vi "checkSettled.vi"(8 "error in (no error)":errorcluster, 11 "Model in":refnum<class "Model.lvclass">) -> (0 "error out":errorcluster, 2 "settledIsTrue":bool, 3 "Model out":refnum<class "Model.lvclass">)   [LabVIEW 2015, in "Model.lvclass"]
uses:
  Model.lvclass
  Model.lvclass/Model.ctl
  ApplicationElements/SystemController/SystemController.lvclass/SystemController.ctl
  ApplicationElements/SystemController/SystemController.lvclass
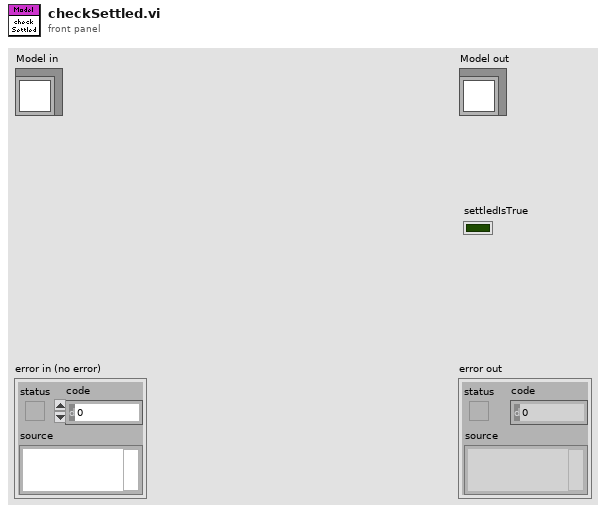
[diagram p1: front panel]
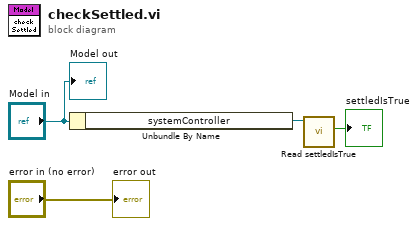
[diagram p0: block diagram]
diagram:
  n1 = Unbundle By Name("Model in") -> ("systemController"=w2:refnum<class "SystemController.lvclass">)
  n2 = call "Read settledIsTrue.vi"("SystemController in"=w2) -> ("settledIsTrue"=→"settledIsTrue":bool)  [unwired: 9 in, 1 out]
  "error out" <- "error in (no error)"
  "Model out" <- "Model in"
